vi "cs-scanning_v3.vi"() -> ()   [LabVIEW 2017]
uses:
  controls/boolean_info.ctl
  controls/z-axis-params_v3.ctl
  <vilib>/rvi/Emulation/niFpgaGetClockAttributes.vi
  <vilib>/rvi/Emulation/niFpgaSctlEmulationGetInTimedLoop.vi
  <vilib>/rvi/Emulation/niFpgaEmulationReportErrorSimple.vi
  <vilib>/rvi/Emulation/niFpgaProcessEmulError.vi
  <vilib>/rvi/eio/common/nirviEmuTemplateMethod_errors.vi
  <vilib>/rvi/Emulation/niFpgaEmulationIsFPGAContextNoSignature.vi
  <vilib>/rvi/DataTransferAndStorage/Container/Common/niFpgaContainerGetUniqueNameForEmu.vi
  <vilib>/rvi/Memory/Memory_Emulation/niFpgaMemoryEmulationCacheClearOnFirstRun.vi
  <vilib>/rvi/Memory/Memory_Emulation/nirvimemoryEmulationManagerCache_MakeExclusive.vi
  <vilib>/rvi/Memory/Memory_Emulation/niFpgaMemoryEmulationValidateCache.vi
  <vilib>/rvi/Memory/Memory_Emulation/nirvimemoryEmulationManagerCache_InsertValue.vi
  <vilib>/Utility/error.llb/Clear Errors.vi
  <vilib>/rvi/Memory/Memory_Emulation/nirvimemoryEmulationManagerCache_ReleaseExclusive.vi
  <vilib>/rvi/Memory/Memory_Emulation/nirvimemoryEmulationManagerCache_GetValue.vi
  <vilib>/rvi/Memory/Memory_Emulation/nirvimemoryEmulationManagerCache_SetValue.vi
  <vilib>/rvi/Emulation/niFpgaCriticalErrorInLSC.vi
  <vilib>/eio/EIONode/EIONode.xnode
  <vilib>/rvi/DataTransferAndStorage/Container/XNode/niFpgaContainer.xnode
  <vilib>/rvi/DataTransferAndStorage/Register/Emulation/niFpgaRegisterEmulation.vi
  FPGA-data-logging.lvlib
  libimaging-cs.lvlib
panel:
  in  "ramp_down":bool
  in  "z_axis_params":T1={"TOL"=0.3, "ramp_rate"=-5e-06, "z_u_max"=5.0, "setpoint"=0.0, "Ki"=0.001, "Z_error_threshold"=0.0, "Z_settled_samples_threshold "=0, "zup_rate"=0.0, "uz_safe"=0.0, "Kiz_down"=0.001, "max_Z_settle_samples"=5000} {"uz_safe" format="%#_13g"; "Z_error_threshold" format="%#_13g"; "ramp_rate" format="%#_4g"; "TOL" format="%#_13g"}
  out "stop_loops":bool
  out "xy_k":fxp<+/-,16,5>[](array[numeric])
  out "xy_ref":fxp<+/-,16,5>[](array[numeric])
  out "u_x saturated":bool
  out "u_y saturated":bool
  out "state1-count":u64
  out "state5-count":u64
  out "state4-count":u64
  out "state3-count":u64
  out "state2-count":u64
  in  "collect all":bool
  out "entity-index":i16
  in  "TsTicks":u32=1600
  out "number-settled-samples-Z":i16
  out "Current Case":u8
  out "boolean \nindicators":T2
  out "z-u(k)":sgl
  in  "ABORT":bool
  out "read fifo timeout":bool
  in  "numEntities":i16
  in  "init Z up":fxp<+/-,16,5>
  in  "trigger-0":bool
  out "number-settled-samples-y":i16
  out "number-settled-samples-x":i16
  in  "xy-error-threshold":sgl format="%#_13g"
  in  "settled-samples\nthreshold":i16
  in  "Ki-xy":sgl=0.001 format="%#_13g"
  in  "xy-bound":sgl
  # "- If collect all = fasle ,\nwe only collect measurement data.\n- If collect all = true, we collect everything."
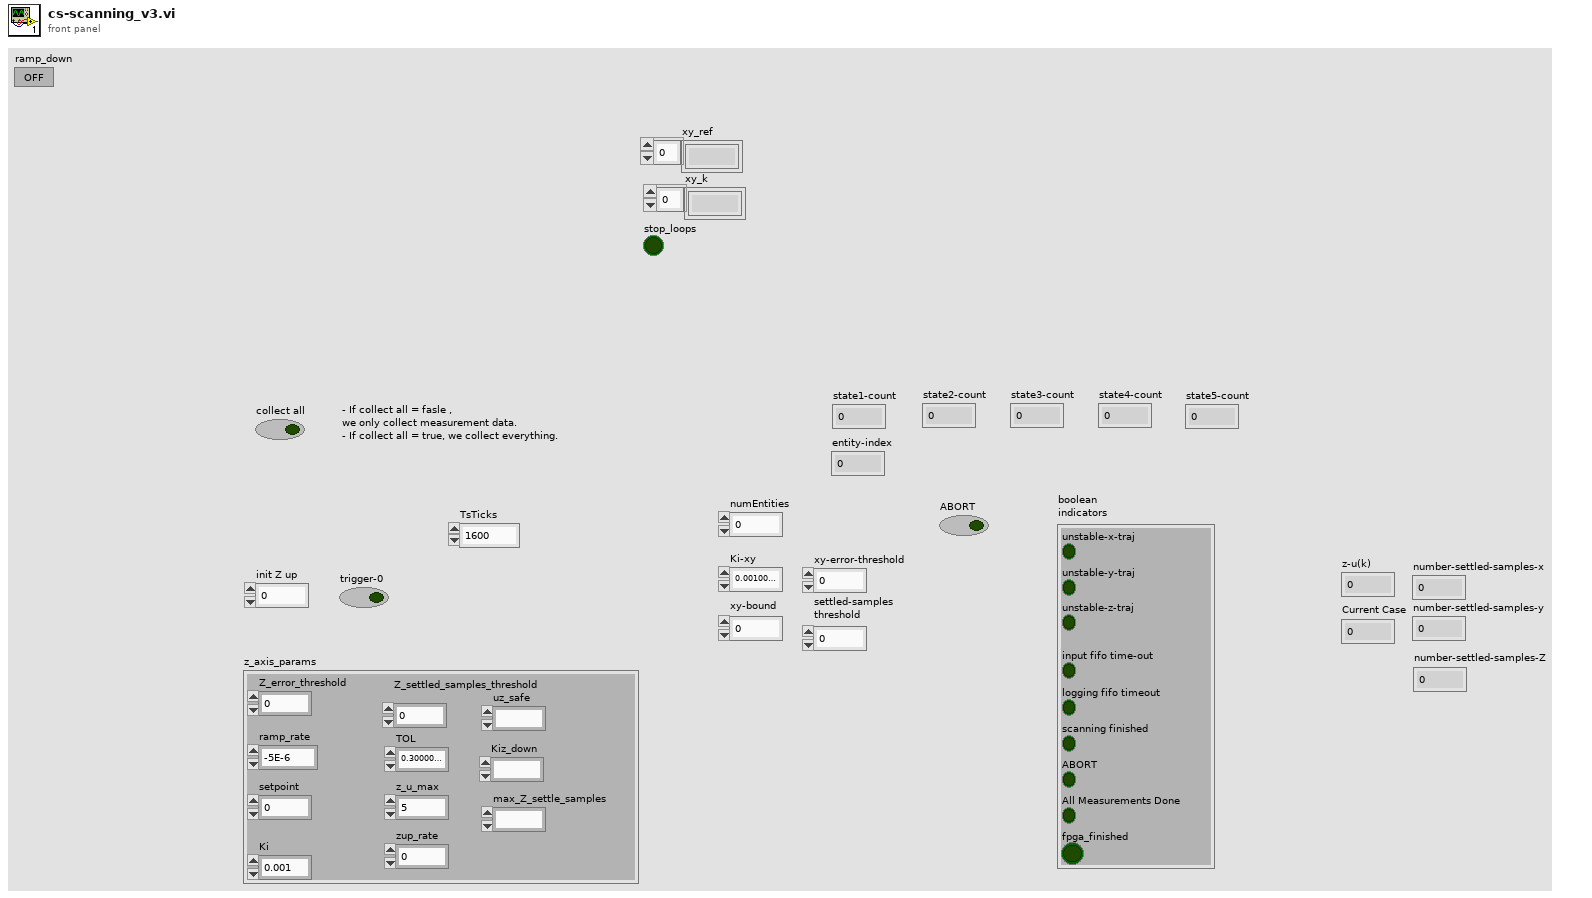
[diagram p1: front panel]
types:
  T1 = typedef "z-axis-params_v3.ctl" = cluster{"TOL":sgl, "ramp_rate":sgl, "z_u_max":sgl, "setpoint":sgl, "Ki":sgl, "Z_error_threshold":sgl, "Z_settled_samples_threshold ":i16, "zup_rate":sgl, "uz_safe":fxp<+/-,16,5>, "Kiz_down":sgl, "max_Z_settle_samples":i16}
  T2 = typedef "boolean_info.ctl" = cluster{"unstable-z-traj":bool, "input fifo time-out":bool, "logging fifo timeout":bool, "scanning finished":bool, "unstable-x-traj":bool, "unstable-y-traj":bool, "ABORT":bool, "All Measurements Done":bool, "fpga_finished":bool}
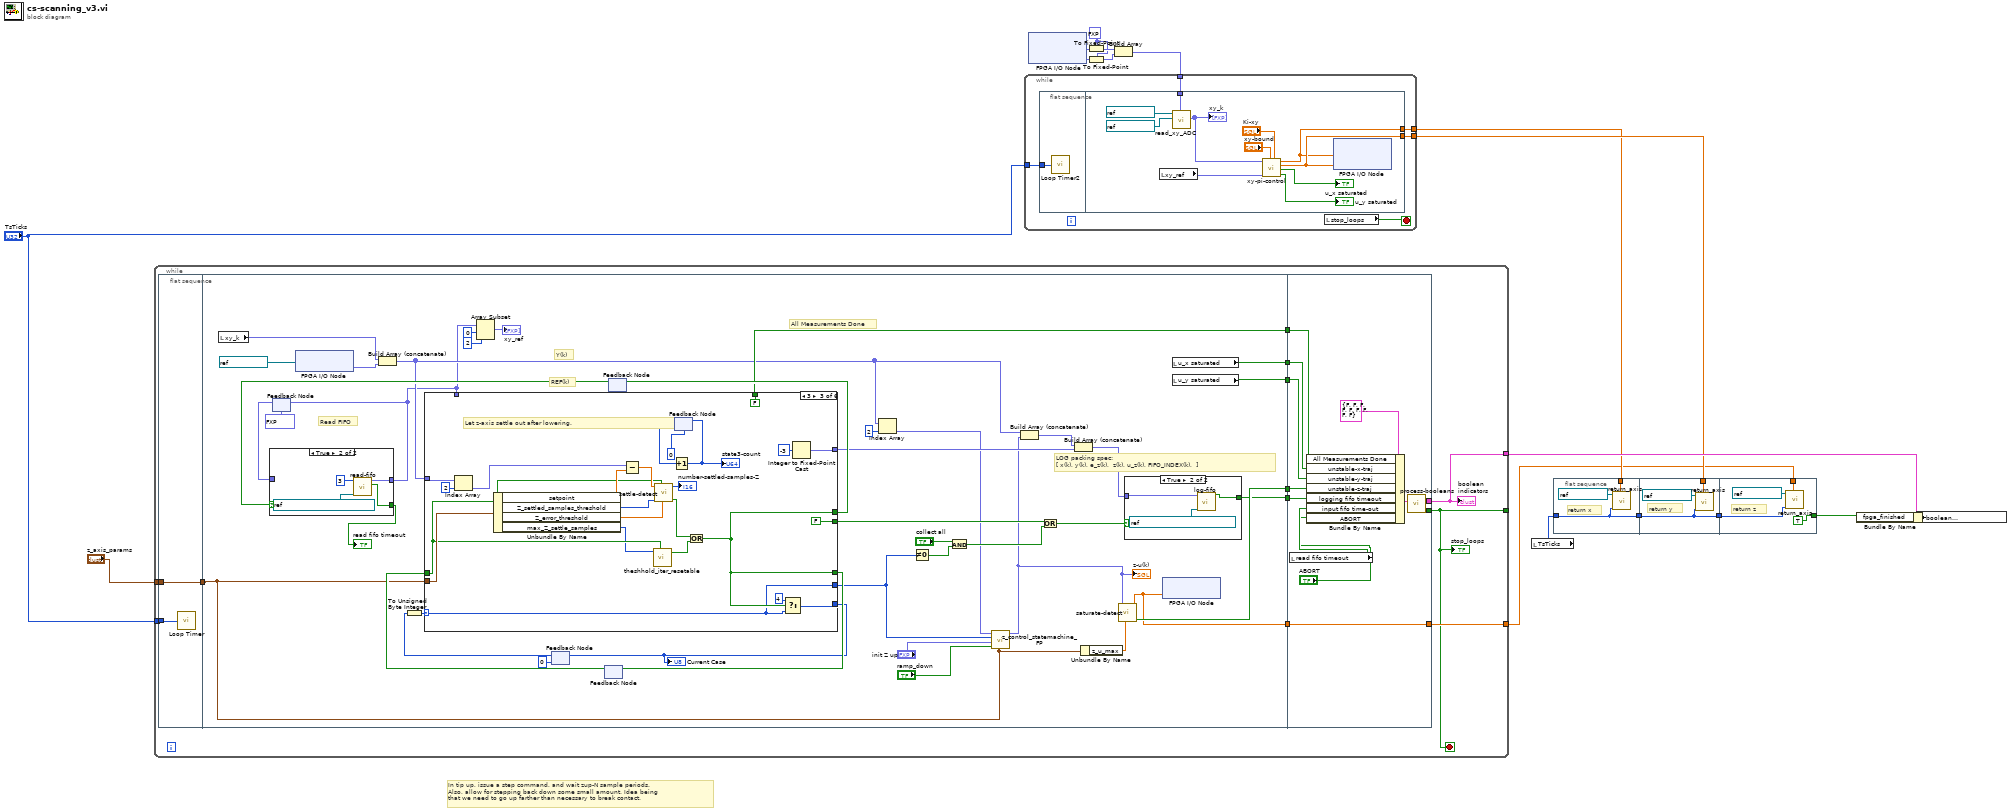
[diagram p0: block diagram]
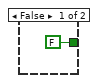
[diagram p2: hidden frame]
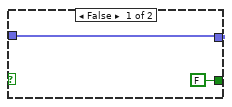
[diagram p3: hidden frame]
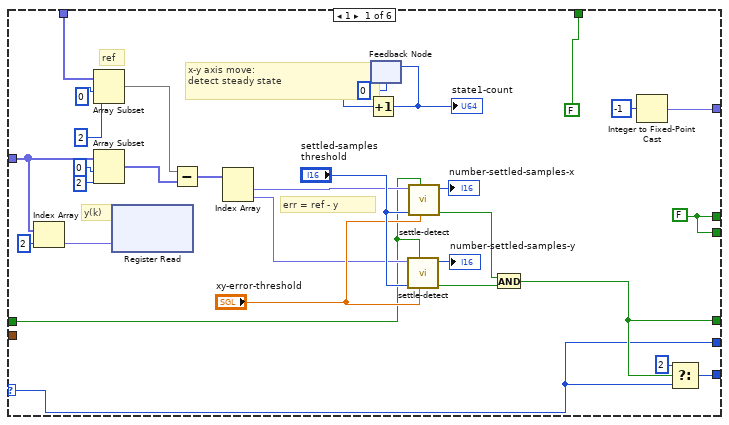
[diagram p4: hidden frame]
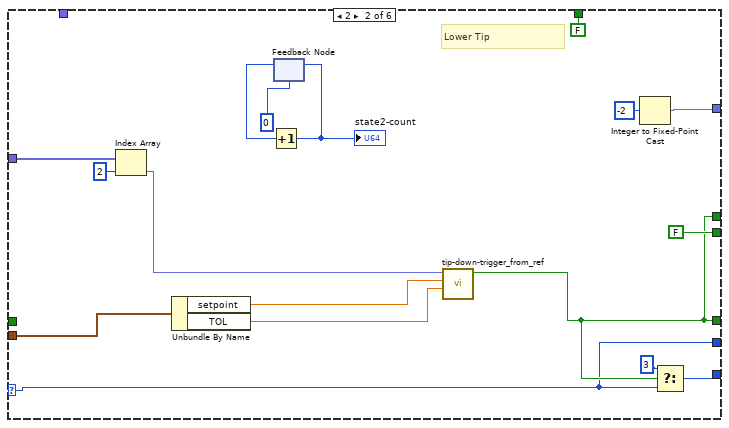
[diagram p5: hidden frame]
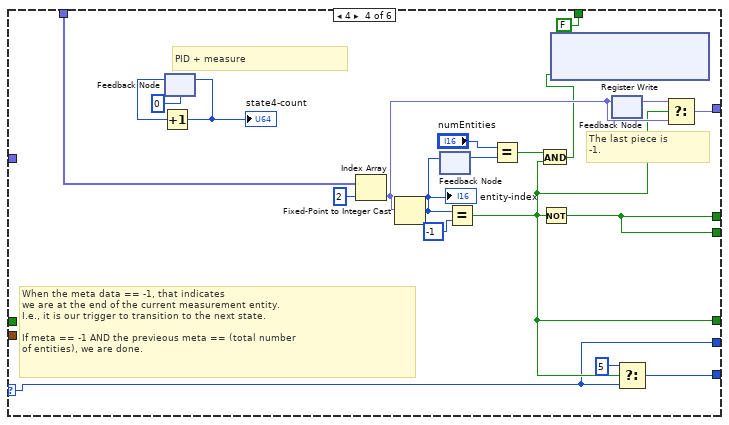
[diagram p6: hidden frame]
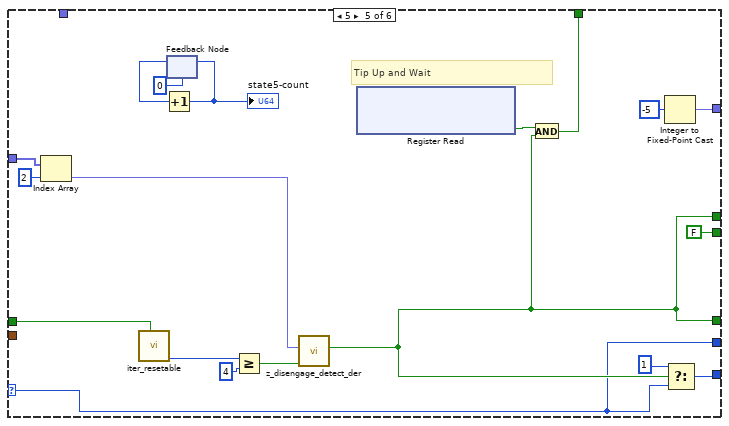
[diagram p7: hidden frame]
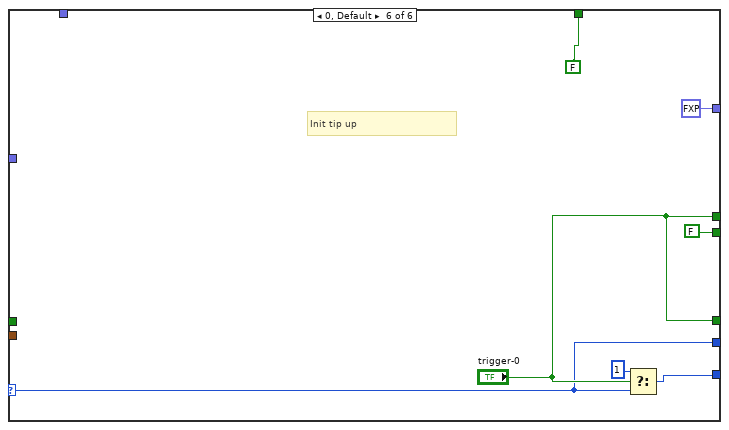
[diagram p8: hidden frame]
diagram:
  w13 = fxp<+/-,16,5> 0.0 ("fixed-point type")
  # "In tip up, issue a step command, and wait zup-N sample periods.\nAlso, allow for stepping back down some small amount. Idea being \nthat we need to go up farther than necessary to break contact."
  n1 = while {
    tunnel: "z_axis_params" -> [w25]
    tunnel: "TsTicks" -> [w24]
    tunnel: [w20] -> _
    tunnel: [w22] -> w2
    tunnel: [w21] -> w9
    stop <- w20 stop-if-true
    n2 = flat-sequence {
      tunnel: w24 -> [w30]
      tunnel: w25 -> [w31]
      tunnel: [w31] -> w29
      tunnel: w29 -> [w40]
      tunnel: [w70] -> w28
      tunnel: [w69] -> w27
      tunnel: [w56] -> w26
      tunnel: [w64] -> w23
      tunnel: [w51] -> w19
      tunnel: [w50] -> w18
      tunnel: w28 -> [w212]
      tunnel: w27 -> [w209]
      tunnel: w26 -> [w206]
      tunnel: [w205] -> w20
      tunnel: [w204] -> w21
      tunnel: [w203] -> w22
      tunnel: w23 -> [w203]
      tunnel: w19 -> [w202]
      tunnel: w18 -> [w201]
      frame #0 {
        n3 = call "Loop Timer"("Count(Ticks)"=w30) -> ()  [unwired: 1 out]
      }
      frame #1 {
        # "All Measurements Done"
        # "REF(k)"
        # "Y(k)"
        # "LOG packing spec:\n[ x(k), y(k), e_z(k),  z(k), u_z(k), FIFO_INDEX(k),  ]"
        # "Read FIFO"
        n4 = local read "xy_k"() -> (w43:fxp<+/-,16,5>[])
        n5 = feedback #1(fxp<+/-,16,5>[] [0.0, 0.0, 0.0] ("unpacked-data")) -> (w72:fxp<+/-,16,5>[])
        n6 = xnode "FPGA I/O Node"("FPGA I/O In"=refnum<k21> "Mod2/AI2" ("y - ADC")) -> ("I/O Item"=w47:fxp<+/-,24,5>)  [unwired: 1 out]
        n7 = Build Array (concatenate)(w43, w47) -> (w46:fxp<+/-,24,5>[])
        n8 = feedback #2(u8 0 ("t")) -> (w41:u8)
        n9 = To Unsigned Byte Integer(number=w41) -> (unsigned 8bit integer=w42:u8)
        n10 = feedback #3() -> (w62:bool)  [unwired: 1 in]
        n11 = feedback #4() -> (w66:bool)  [unwired: 1 in]
        n12 = case shown="True" w66 {
          tunnel: w72 -> [w78 _]
          tunnel: [w78 w80] -> w32
          tunnel: [FALSE ("timout?") w79] -> w68
          frame False {
          }
          frame True {
            n13 = call "read-fifo.vi"("FIFO In"=refnum<k21> "host-to-fpga-fxp-16-5", "numChan"=3) -> ("timout?"=w79:bool, "unpacked-data"=w80:fxp<+/-,16,5>[])  [unwired: 8 in]
          }
        }
        "read fifo timeout" <- w68
        n14 = feedback-in #1(w32) -> ()
        n15 = case shown="3" w42 {
          selector: w42 -> [w83 w114 w132 w155 w175 w194]
          tunnel: [w84 FALSE FALSE ("trigger-0") w165 FALSE FALSE] -> w57
          tunnel: [w106 w126 w148 w173 w192 w200] -> w38
          tunnel: w46 -> [w85 w128 w152 _ w183 _]
          tunnel: [w84 w116 w135 w165 w178 "trigger-0"] -> w67
          tunnel: w40 -> [_ w130 w146 _ _ _]
          tunnel: [FALSE FALSE FALSE FALSE w185 FALSE] -> w56
          tunnel: w32 -> [w97 _ _ w167 _ _]
          tunnel: w62 -> [w95 _ w133 _ w177 _]
          tunnel: [w94 w116 w135 w158 w178 "trigger-0"] -> w63
          tunnel: [w88 w117 w138 w161 w186 fxp<+/-,16,5> 0.0 ("Element")] -> w44
          tunnel: [w83 w114 w132 w155 w175 w194] -> w33
          frame 1 {
            w84 = FALSE
            # "y(k)"
            # "err = ref - y"
            # "ref"
            # "x-y axis move: \ndetect steady state"
            n16 = Index Array(array=w85, index=2) -> (element=w87:fxp<+/-,24,5>)
            n17 = Array Subset(array=w97, index=0, length=2) -> (w101:fxp<+/-,16,5>[])
            n18 = Array Subset(array=w85, index=0, length=2) -> (w100:fxp<+/-,24,5>[])
            n19 = xnode ("Register Read")("Data"=w87) -> ()  [unwired: 1 in, 1 out]
            n20 = Subtract(x=w101, y=w100) -> (x-y=w93:fxp<+/-,25,6>[])
            n21 = Index Array(array=w93) -> (element #1=w99:fxp<+/-,25,6>, element #2=w98:fxp<+/-,25,6>)  [unwired: 2 in]
            n22 = feedback #5(u64 0) -> (w91:u64)
            n23 = Increment(x=w91) -> (x+1=w92:u64)
            "state1-count" <- w92
            n24 = feedback-in #5(w92) -> ()
            n25 = call "settle-detect.vi"("error-max"="xy-error-threshold", "reset"=w95, "settled-samples\nthreshold"="settled-samples\nthreshold", "err(k)"=w98) -> ("has-settled"=w113:bool, "number-settled-samples"=→"number-settled-samples-y":u16)  [unwired: 6 in]
            n26 = call "settle-detect.vi"("error-max"="xy-error-threshold", "reset"=w95, "settled-samples\nthreshold"="settled-samples\nthreshold", "err(k)"=w99) -> ("has-settled"=w112:bool, "number-settled-samples"=→"number-settled-samples-x":u16)  [unwired: 6 in]
            n27 = And(x=w112, y=w113) -> (x .and. y?=w94:bool)
            n28 = Integer to Fixed-Point Cast(integer=i16 -1) -> (fixed-point=w88:fxp<+/-,16,5>)  [unwired: 1 in]
            n29 = Select(t=u8 2, s=w94, f=w83) -> (s? t:f=w106:u8)
          }
          frame 2 {
            # "Lower Tip"
            n30 = Index Array(array=w128, index=2) -> (element=w127:fxp<+/-,24,5>)
            n31 = Unbundle By Name(w130) -> ("setpoint"=w118:sgl, "TOL"=w115:sgl)
            n32 = feedback #6(u64 0) -> (w121:u64)
            n33 = Increment(x=w121) -> (x+1=w122:u64)
            "state2-count" <- w122
            n34 = feedback-in #6(w122) -> ()
            n35 = call "tip-down-trigger_from_ref.vi"("TOL"=w115, "setpoint"=w118, "I/O Item"=w127) -> ("Boolean"=w116:bool)  [unwired: 8 in]
            n36 = Integer to Fixed-Point Cast(integer=i16 -2) -> (fixed-point=w117:fxp<+/-,16,5>)  [unwired: 1 in]
            n37 = Select(t=u8 3, s=w116, f=w114) -> (s? t:f=w126:u8)
          }
          frame 3 {
            # "Let z-axis settle out after lowering."
            n38 = Index Array(array=w152, index=2) -> (element=w150:fxp<+/-,24,5>)
            n39 = Unbundle By Name(w146) -> ("setpoint"=w137:sgl, "Z_settled_samples_threshold"=w145:i16, "Z_error_threshold"=w144:sgl, "max_Z_settle_samples"=w131:i16)
            n40 = Subtract(x=w150, y=w137) -> (x-y=w153:sgl)
            n41 = call "theshhold_iter_resetable.vi"("reset"=w133, "N"=w131) -> ("Boolean"=w134:bool)  [unwired: 8 in, 1 out]
            n42 = call "settle-detect.vi"("error-max"=w144, "reset"=w133, "settled-samples\nthreshold"=w145, "err(k)"=w153) -> ("has-settled"=w136:bool, "number-settled-samples"=→"number-settled-samples-Z":u16)  [unwired: 6 in]
            n43 = feedback #7(u64 0) -> (w141:u64)
            n44 = Increment(x=w141) -> (x+1=w142:u64)
            "state3-count" <- w142
            n45 = feedback-in #7(w142) -> ()
            n46 = Or(x=w136, y=w134) -> (x .or. y?=w135:bool)
            n47 = Select(t=u8 4, s=w135, f=w132) -> (s? t:f=w148:u8)
            n48 = Integer to Fixed-Point Cast(integer=i16 -3) -> (fixed-point=w138:fxp<+/-,16,5>)  [unwired: 1 in]
          }
          frame 4 {
            # "The last piece is\n-1."
            # "When the meta data == -1, that indicates\nwe are at the end of the current measurement entity.\nI.e., it is our trigger to transition to the next state.\n\nIf meta == -1 AND the previeous meta == (total number\nof entities), we are done."
            # "PID + measure"
            n49 = feedback #8(u64 0) -> (w163:u64)
            n50 = Increment(x=w163) -> (x+1=w164:u64)
            "state4-count" <- w164
            n51 = feedback-in #8(w164) -> ()
            n52 = Index Array(array=w167, index=2) -> (element=w159:fxp<+/-,16,5>)
            n53 = Fixed-Point to Integer Cast(1:w159) -> (0:w166:i16)
            "entity-index" <- w166
            n54 = feedback #9() -> (w168:i16)  [unwired: 1 in]
            n55 = feedback-in #9(w166) -> ()
            n56 = Equal?(x=w166, y=i16 -1) -> (x = y?=w158:bool)
            n57 = Equal?(x="numEntities", y=w168) -> (x = y?=w169:bool)
            n58 = And(x=w169, y=w158) -> (x .and. y?=w157:bool)
            n59 = Not(x=w158) -> (.not. x?=w165:bool)
            n60 = xnode ("Register Write")("Data"=w157) -> ()  [unwired: 1 in, 1 out]
            n61 = feedback #10() -> (w160:fxp<+/-,16,5>)  [unwired: 1 in]
            n62 = feedback-in #10(w159) -> ()
            n63 = Select(t=u8 5, s=w158, f=w155) -> (s? t:f=w173:u8)
            n64 = Select(t=w160, s=w158, f=w159) -> (s? t:f=w161:fxp<+/-,16,5>)
          }
          frame 5 {
            # "Tip Up and Wait"
            n65 = Index Array(array=w183, index=2) -> (element=w182:fxp<+/-,24,5>)
            n66 = call "iter_resetable.vi"("reset"=w177) -> ("iter"=w176:i16)  [unwired: 10 in]
            n67 = feedback #11(u64 0) -> (w189:u64)
            n68 = Increment(x=w189) -> (x+1=w190:u64)
            "state5-count" <- w190
            n69 = feedback-in #11(w190) -> ()
            n70 = Greater Or Equal?(x=w176, y=i16 4) -> (x >= y?=w181:bool)
            n71 = call "z_disengage_detect_der.vi"("start_der_calc"=w181, "z_err"=w182) -> ("z_has_disengaged"=w178:bool)  [unwired: 9 in]
            n72 = xnode ("Register Read")() -> ("Data"=w179:bool)  [unwired: 1 in, 1 out]
            n73 = And(x=w179, y=w178) -> (x .and. y?=w185:bool)
            n74 = Integer to Fixed-Point Cast(integer=i16 -5) -> (fixed-point=w186:fxp<+/-,16,5>)  [unwired: 1 in]
            n75 = Select(t=u8 1, s=w178, f=w175) -> (s? t:f=w192:u8)
          }
          frame 0, Default {
            # "Init tip up"
            n76 = Select(t=u8 1, s="trigger-0", f=w194) -> (s? t:f=w200:u8)
          }
        }
        "Current Case" <- w38
        n77 = Array Subset(array=w32, index=0, length=2) -> (→"xy_ref":fxp<+/-,16,5>[])
        n78 = feedback-in #2(w38) -> ()
        n79 = feedback-in #3(w63) -> ()
        n80 = feedback-in #4(w67) -> ()
        n81 = Index Array(array=w46, index=2) -> (element=w37:fxp<+/-,24,5>)
        n82 = Not Equal To 0?(x=w33) -> (x != 0?=w60:bool)
        n83 = And(x="collect all", y=w60) -> (x .and. y?=w58:bool)
        n84 = call "z_control_statemachine_FP.vi"("z_axis_params"=w40, "ramp_down"="ramp_down", "init Z up"="init Z up", "State"=w33, "zerr(k)"=w37) -> ("z-u(k)"=w39:fxp<+/-,16,5>)  [unwired: 6 in]
        "z-u(k)" <- w39
        n85 = Build Array (concatenate)(w46, w39) -> (w45:fxp<+/-,24,5>[])
        n86 = Or(x=w57, y=w58) -> (x .or. y?=w61:bool)
        n87 = Build Array (concatenate)(w45, w44) -> (w71:fxp<+/-,24,5>[])
        n88 = Unbundle By Name(w40) -> ("z_u_max"=w54:sgl)
        n89 = call "saturate-detect.vi"("bound"=w54, "x"=w39) -> ("saturated"=w70:bool, "sat(x)"=w64:sgl)  [unwired: 8 in]
        n90 = case shown="True" w61 {
          tunnel: w71 -> [_ w75]
          tunnel: [FALSE ("logging-timeout?") w74] -> w69
          frame False {
          }
          frame True {
            n91 = call "log-fifo.vi"("FIFO In"=refnum<k21> "fpga-to-host2-fxp-16-5", "input-data"=w75) -> ("logging-timeout?"=w74:bool)  [unwired: 9 in]
          }
        }
        n92 = xnode "FPGA I/O Node"("Mod1/AO2"=w64) -> ()  [unwired: 1 in, 1 out]
        n93 = local read "u_x saturated"() -> (w51:bool)
        n94 = local read "u_y saturated"() -> (w50:bool)
      }
      frame #2 {
        n95 = local read "read fifo timeout"() -> (w208:bool)
        n96 = Bundle By Name(cluster=T2 {"unstable-z-traj"=FALSE, "input fifo time-out"=FALSE, "logging fifo timeout"=FALSE, "scanning finished"=FALSE, "unstable-x-traj"=FALSE, "unstable-y-traj"=FALSE, "ABORT"=FALSE, "All Measurements Done"=FALSE, "fpga_finished"=FALSE} ("boolean errors"), "All Measurements Done"=w206, "unstable-x-traj"=w202, "unstable-y-traj"=w201, "unstable-z-traj"=w212, "logging fifo timeout"=w209, "input fifo time-out"=w208, "ABORT"="ABORT") -> (w210:T2)
        n97 = call "process-booleans.vi"("boolean indicators 2"=w210) -> ("scaning finished"=w205:bool, "boolean indicators"=w204:T2)  [unwired: 9 in]
      }
    }
    "boolean \nindicators" <- w21
    "stop_loops" <- w20
  }
  n98 = xnode "FPGA I/O Node"() -> ("Mod2/AI0"=w16:fxp<+/-,24,5>, "Mod2/AI1"=w14:fxp<+/-,24,5>)  [unwired: 2 in, 2 out]
  n99 = To Fixed-Point(fixed-point type=w13, number=w16) -> (fixed-point=w17:fxp<+/-,16,5>)
  n100 = To Fixed-Point(fixed-point type=w13, number=w14) -> (fixed-point=w15:fxp<+/-,16,5>)
  n101 = Build Array(w17, w15) -> (w3:fxp<+/-,16,5>[])
  n102 = while {
    tunnel: "TsTicks" -> [w217]
    tunnel: [w216] -> w5
    tunnel: [w215] -> w4
    tunnel: w3 -> [w214]
    stop <- w213 stop-if-true
    n103 = flat-sequence {
      tunnel: w217 -> [w218]
      tunnel: [w228] -> w216
      tunnel: [w227] -> w215
      tunnel: w214 -> [w223]
      frame #0 {
        n104 = call "Loop Timer2"("Count(Ticks)"=w218) -> ()  [unwired: 1 out]
      }
      frame #1 {
        n105 = local read "xy_ref"() -> (w220:fxp<+/-,16,5>[])
        n106 = call "read_xy_ADC.vi"("x(0), y(0)"=w223, "y - ADC"=refnum<k21> "Mod2/AI1", "x - ADC"=refnum<k21> "Mod2/AI0") -> ("x_y"=w219:fxp<+/-,17,6>[])  [unwired: 8 in]
        "xy_k" <- w219
        n107 = call "xy-pi-control.vi"("Ki-xy"="Ki-xy", "xy-umax"="xy-bound", "xy-ref"=w220, "x_k-y_k"=w219) -> ("u_y saturated"=→"u_y saturated":bool, "u_x saturated"=→"u_x saturated":bool, "sat(u_y)"=w228:sgl, "sat(u_x)"=w227:sgl)  [unwired: 4 in]
        n108 = xnode "FPGA I/O Node"("Mod1/AO0"=w227, "Mod1/AO1"=w228) -> ()  [unwired: 2 in, 2 out]
      }
    }
    n109 = local read "stop_loops"() -> (w213:bool)
  }
  n110 = local read "TsTicks"() -> (w10:u32)
  n111 = flat-sequence {
    tunnel: w10 -> [w231]
    tunnel: w4 -> [w232]
    tunnel: [w231] -> w12
    tunnel: w5 -> [w235]
    tunnel: w12 -> [w233]
    tunnel: [w233] -> w11
    tunnel: w2 -> [w239]
    tunnel: w11 -> [w237]
    tunnel: [TRUE] -> w8
    frame #0 {
      # "return x"
      n112 = call "return_axis.vi"("u(0)"=w232, "TsTicks"=w231, "FPGA I/O In"=refnum<k21> "Mod1/AO0") -> ()  [unwired: 9 in]
    }
    frame #1 {
      # "return y"
      n113 = call "return_axis.vi"("u(0)"=w235, "TsTicks"=w233, "FPGA I/O In"=refnum<k21> "Mod1/AO1") -> ()  [unwired: 9 in]
    }
    frame #2 {
      # "return z"
      n114 = call "return_axis.vi"("u(0)"=w239, "TsTicks"=w237, "FPGA I/O In"=refnum<k21> "Mod1/AO2") -> ()  [unwired: 9 in]
    }
  }
  n115 = Bundle By Name(cluster=w9, "fpga_finished"=w8) -> (w7:T2)
  n116 = local write "boolean \nindicators"(w7) -> ()
